vi "No Request Remaining.vi"(8 "error in (no error)":errorcluster, 11 "Elevator Controller in":refnum<class "Elevator Controller.lvclass">) -> (0 "error out":errorcluster, 3 "Elevator Controller out":refnum<class "Elevator Controller.lvclass">)   [LabVIEW 2019]
uses:
  Elevator Controller.lvclass
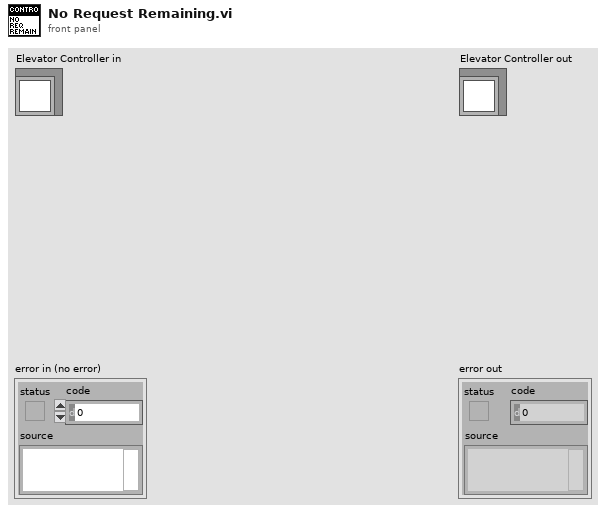
[diagram p1: front panel]
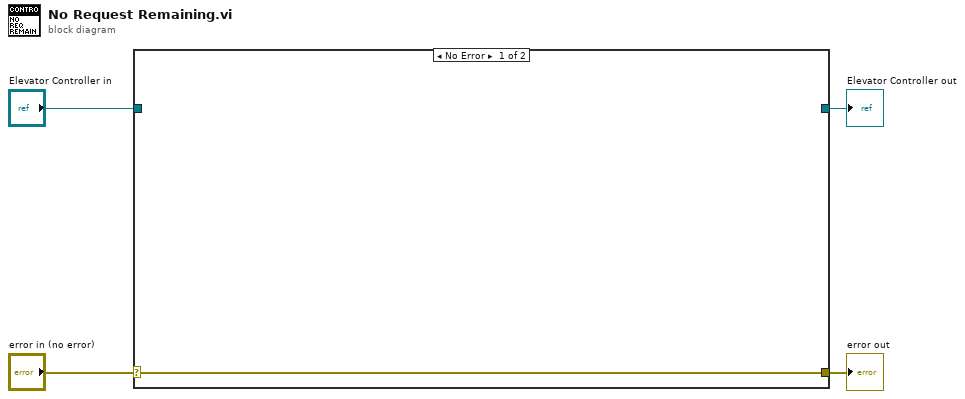
[diagram p0: block diagram]
diagram:
  n1 = case shown="No Error" "error in (no error)" {
    selector: "error in (no error)" -> [w5 w7]
    tunnel: [w5 w7] -> w3
    tunnel: [_ w6] -> w1
    tunnel: "Elevator Controller in" -> [_ w6]
    frame No Error {
    }
    frame Error {
    }
  }
  "error out" <- w3
  "Elevator Controller out" <- w1
